vi "Dialog_LoadFile.vi"() -> (3 "LoadAction OUT":enum32{"SameDir", "Copy", "Cancel"}(ring))   [LabVIEW 2012]
doc: "This is the dialog window allowing user to select the action to be performed on selecting the Load Option"
panel:
  in  "Cancel":bool
  in  "OK":bool
  in  "LoadAction":enum32{"SameDir", "Copy"}(radio)
  # "Please select the required action"
  # "(The selected file will be opened for editing)"
  # "(Additional copy of the selected file will be created for editing. The original file will be unaltered)"
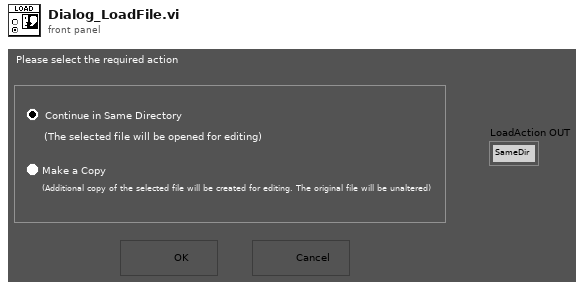
[diagram p1: front panel]
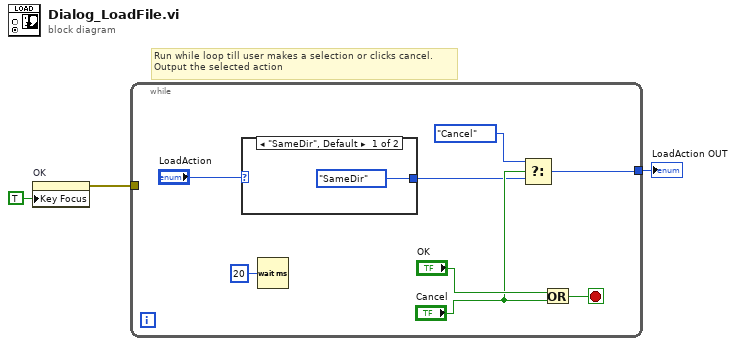
[diagram p0: block diagram]
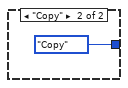
[diagram p2: hidden frame]
diagram:
  # "Run while loop till user makes a selection or clicks cancel.\nOutput the selected action"
  n1 = property on="OK" class="Bool"("Key Focus"=TRUE) -> (error out=w1:errorcluster)  [unwired: 2 in, 1 out]
  n2 = while {
    tunnel: [w5] -> w3
    tunnel: w1 -> [_]
    stop <- w10 stop-if-true
    n3 = case shown="\"SameDir\", Default" "LoadAction" {
      tunnel: [enum32{"SameDir", "Copy", "Cancel"}."SameDir" ("LoadAction") enum32{"SameDir", "Copy", "Cancel"}."Copy" ("LoadAction")] -> w6
      frame "SameDir", Default {
      }
      frame "Copy" {
      }
    }
    n4 = Wait (ms)(milliseconds to wait=u32 20) -> ()  [unwired: 1 out]
    n5 = Select(t=enum32{"SameDir", "Copy", "Cancel"}."Cancel" ("LoadAction"), s="Cancel", f=w6) -> (s? t:f=w5:enum32{"SameDir", "Copy", "Cancel"})
    n6 = Or(x="OK", y="Cancel") -> (x .or. y?=w10:bool)
  }
  "LoadAction OUT" <- w3
